vi "Set Position Enabled.vi"(8 "error in (no error)":errorcluster, 10 "Position Enabled":bool, 11 "Team Config Panel in":refnum<class "Team Config Panel.lvclass">) -> (0 "error out":errorcluster, 3 "Team Config Panel out":refnum<class "Team Config Panel.lvclass">)   [LabVIEW 2020, in "SB App.lvlib" / "Team Config Panel.lvclass"]
uses:
  Team Config Panel.lvclass
  Position Enabled Data.ctl
  Team Config Panel.lvclass/Team Config Panel.ctl
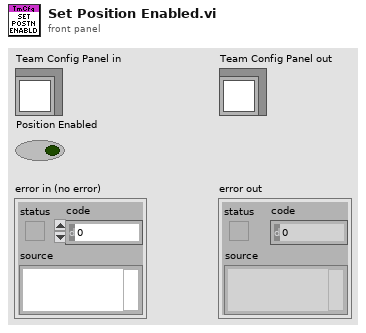
[diagram p1: front panel]
types:
  T1 = typedef "SB App.lvlib/Team Config Panel.lvclass/Position Enabled Data.ctl" = cluster{"Enabled":bool}
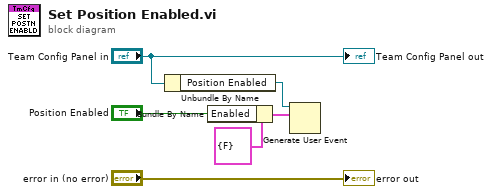
[diagram p0: block diagram]
diagram:
  n1 = Unbundle By Name("Team Config Panel in") -> ("Position Enabled"=w4:refnum<user-event>)
  n2 = Bundle By Name(cluster=T1 {"Enabled"=FALSE} ("event data"), "Enabled"="Position Enabled") -> (w2:T1)
  n3 = Generate User Event(user event=w4, event data cluster=w2) -> ()  [unwired: 2 in, 2 out]
  "error out" <- "error in (no error)"
  "Team Config Panel out" <- "Team Config Panel in"
